vi "Falling Edge Trigger.vi"(1 "Signal":bool) -> (0 "Trigger?":bool)   [LabVIEW 2015]
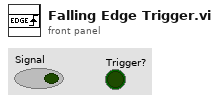
[diagram p1: front panel]
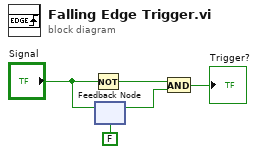
[diagram p0: block diagram]
diagram:
  n1 = Not(x="Signal") -> (.not. x?=w2:bool)
  n2 = feedback #1(FALSE ("Signal")) -> (w1:bool)
  n3 = feedback-in #1("Signal") -> ()
  n4 = And(x=w2, y=w1) -> (x .and. y?=→"Trigger?":bool)
